vi "subComputeConfigPagePath.vi"(9 "Config page path":path, 11 "Class path":path) -> (3 "Path out":path)   [LabVIEW 2020, in "UserInterface.lvlib" / "UIManager.lvclass"]
uses:
  UIManager.lvclass
  CommonHelpers/CommonHelpers.lvlib
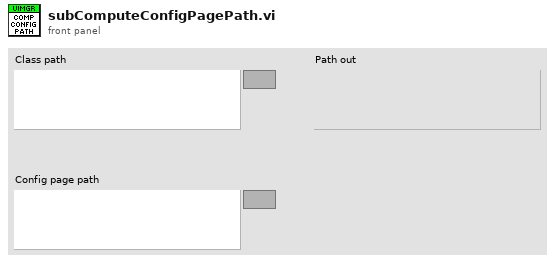
[diagram p1: front panel]
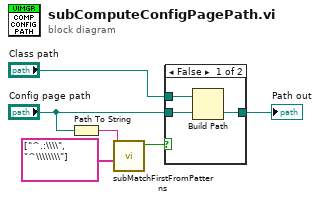
[diagram p0: block diagram]
diagram:
  n1 = Path To String(path="Config page path") -> (string=w6:string)
  n2 = call "subMatchFirstFromPatterns.vi"("patterns"=string[] ["^.:\\\\", "^\\\\\\\\"], "string in"=w6) -> ("found?"=w4:bool)  [unwired: 7 in, 2 out]
  n3 = case shown="False" w4 {
    tunnel: "Config page path" -> [w8 w10]
    tunnel: "Class path" -> [w9 _]
    tunnel: [w7 w10] -> w1
    frame False {
      n4 = Build Path(base path=w9, name or relative path=w8) -> (appended path=w7:path)
    }
    frame True {
    }
  }
  "Path out" <- w1
